vi "Create Group.vi"(8 "name":string, 10 "loc_id":i32, 11 "error in (no error)":errorcluster) -> (2 "group_id":i32, 3 "error out":errorcluster)   [LabVIEW 2010]
uses:
  Release/HDF5Tools.dll
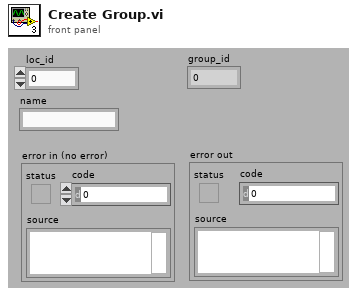
[diagram p1: front panel]
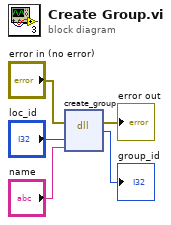
[diagram p0: block diagram]
diagram:
  n1 = dll-call lib="Z:/users/alex/projects/HDF5Tools/Release/HDF5Tools.dll" fn="create_group"(error in="error in (no error)", "loc_id"="loc_id", "name"="name") -> (error out=→"error out":errorcluster, "group_id"=→"group_id":i32)  [unwired: 4 in, 1 out]
